vi "roboRIO v1.0 Get Scaling Constants AO.vi"(8 "error in (no error)":errorcluster, 10 "Channel List":T3) -> (0 "error out":errorcluster, 2 "Scale Constants Array":T1)   [LabVIEW 2021]
uses:
  <vilib>/myRIO/Common/Instrument Driver Framework/myRIO v1.0/AO/typedefs/AO Channels List.ctl
  <vilib>/myRIO/Common/Instrument Driver Framework/myRIO v1.0/AO/typedefs/AO Channels Enum.ctl
  <vilib>/myRIO/Common/Instrument Driver Framework/Utilities/typedefs/Analog Scaling Constants List.ctl
  <vilib>/myRIO/Common/Instrument Driver Framework/Utilities/typedefs/Analog Scaling Constants.ctl
  <vilib>/myRIO/Common/Instrument Driver Framework/roboRIO v1.0/Resource Manager/vis/roboRIO v1.0 Get Scaling Constants.vi
  <vilib>/myRIO/Common/Instrument Driver Framework/Utilities/vis/Parse Scaling Constant Table.vi
  <vilib>/myRIO/Common/Instrument Driver Framework/roboRIO v1.0/Resource Manager/vis/roboRIO v1.0 Scaling Constants Table.vi
  <vilib>/Utility/error.llb/Trim Whitespace.vi
  <vilib>/Utility/error.llb/Error Cluster From Error Code.vi
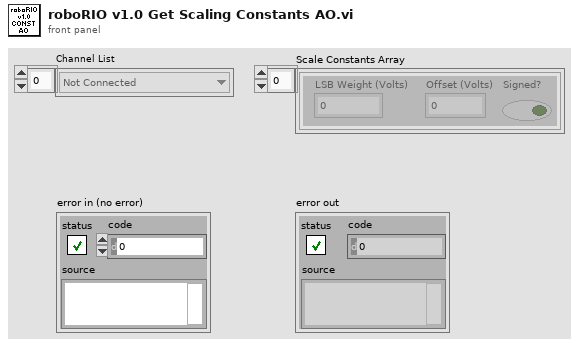
[diagram p1: front panel]
types:
  T1 = typedef "Analog Scaling Constants List.ctl" = T2[]
  T2 = typedef "Analog Scaling Constants.ctl" = cluster{"LSB Weight (Volts)":dbl, "Offset (Volts)":dbl, "Signed?":bool}
  T3 = typedef "AO Channels List.ctl" = T4[]
  T4 = typedef "AO Channels Enum.ctl" = enum16{"Not Connected", "AudioOut/Left", "AudioOut/Right", "C/AO0", "C/AO1", "A/AO0", "A/AO1", "B/AO0", "B/AO1"}
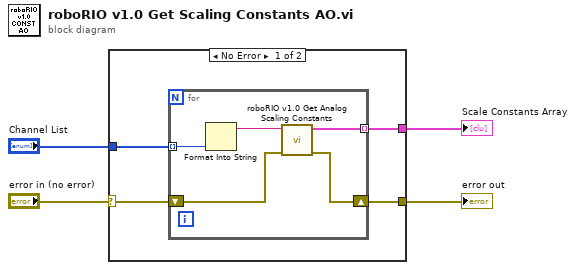
[diagram p0: block diagram]
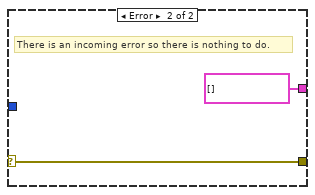
[diagram p2: hidden frame]
diagram:
  n1 = case shown="No Error" "error in (no error)" {
    selector: "error in (no error)" -> [w7 w15]
    tunnel: [w6 w15] -> w2
    tunnel: "Channel List" -> [w8 _]
    tunnel: [w5 T2[] []] -> w1
    frame No Error {
      n2 = for {
        tunnel: w8 -> [w10] mode=indexing
        shift-right: [w11] -> w6
        shift-left: w7 -> [w12]
        tunnel: [w13] -> w5 mode=indexing
        n3 = Format Into String(w10) -> (resulting string=w9:string)  [unwired: 3 in, 1 out]
        n4 = call <vilib>:"roboRIO v1.0 Get Analog Scaling Constants.vi"("error in (no error)"=w12, "Analog Channel Name"=w9) -> ("error out"=w11:errorcluster, "Analog Scaling Constants"=w13:T2)  [unwired: 8 in]
      }
    }
    frame Error {
      # "There is an incoming error so there is nothing to do."
    }
  }
  "error out" <- w2
  "Scale Constants Array" <- w1
